vi "Compute_CheckSum.vi"(8 "error in (no error)":errorcluster, 10 "Trama IN":string) -> (0 "error out":errorcluster, 1 "Checksum ASCII":string="T")   [LabVIEW 2014, in "CAP-USB.lvlib"]
doc: "Ejecuta la operacion de suma \ncorrespondiente al Checksum"
uses:
  CAP-USB.lvlib
panel:
  out "sum":u8
  out "Numeric Values":u8[](array[numeric])
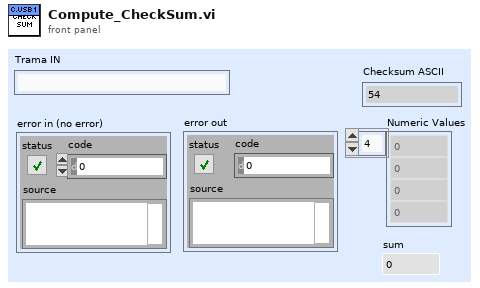
[diagram p1: front panel]
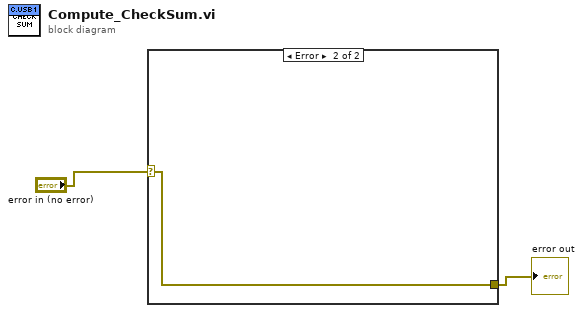
[diagram p0: block diagram]
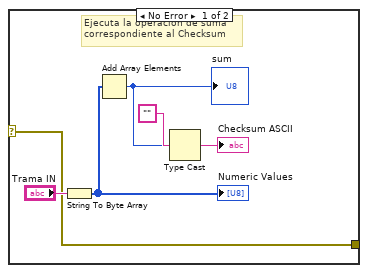
[diagram p2: hidden frame]
diagram:
  n1 = case shown="Error" "error in (no error)" {
    selector: "error in (no error)" -> [w3 w9]
    tunnel: [w3 w9] -> w1
    frame No Error {
      # "Ejecuta la operacion de suma \ncorrespondiente al Checksum"
      n2 = String To Byte Array(string="Trama IN") -> (unsigned byte array=w5:u8[])
      "Numeric Values" <- w5
      n3 = Add Array Elements(numeric array=w5) -> (sum=w4:u8)
      "sum" <- w4
      n4 = Type Cast(type="", x=w4) -> (*(type *) &x=→"Checksum ASCII":string)
    }
    frame Error {
    }
  }
  "error out" <- w1
